vi "recursively populate tree ctl.vi"(8 "error in (no error)":errorcluster, 10 "tree ctl ref":refnum<vi>, 11 "Object path":string="IndivITX/Test1/SA03008N.20190801.000000.itx") -> (0 "error out":errorcluster, 2 "reference out":refnum<vi>)   [LabVIEW 2020, in "Data.S3.lvclass"]
uses:
  Data.S3.lvclass
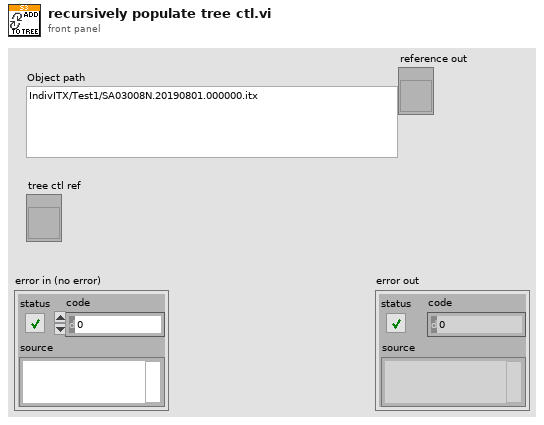
[diagram p1: front panel]
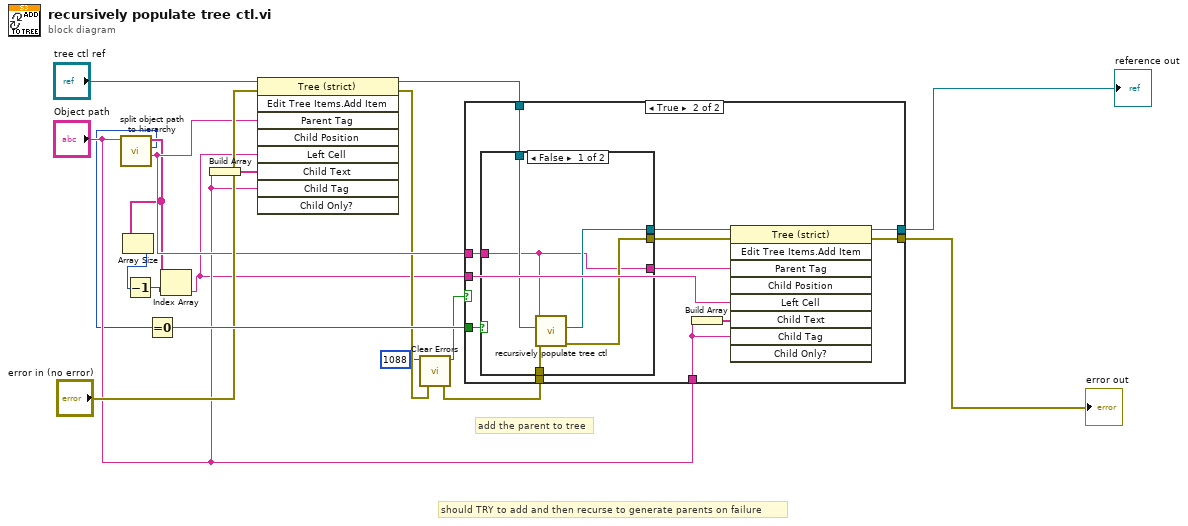
[diagram p0: block diagram]
diagram:
  # "should TRY to add and then recurse to generate parents on failure"
  # "add the parent to tree"
  n1 = call "split object path to hierarchy.vi"("Object path"="Object path") -> ("parent path"=w15:string, "layers"=w2:i32, "hierarchy"=w5:string[])  [unwired: 8 in]
  n2 = Array Size(array=w5) -> (size(s)=w3:i32)
  n3 = Decrement(x=w3) -> (x-1=w4:i32)
  n4 = Equal To 0?(x=w2) -> (x = 0?=w18:bool)
  n5 = Index Array(array=w5, index=w4) -> (element=w1:string)
  n6 = Build Array("Object path") -> (w14:string[])
  n7 = invoke on="Invoke Node" class="Tree (strict)" method="Edit Tree Items.Add Item"(reference="tree ctl ref", error in="error in (no error)", "Parent Tag"=w15, "Left Cell"=w1, "Child Text"=w14, "Child Tag"="Object path") -> (reference out=w12:refnum<vi>, error out=w10:errorcluster)  [unwired: 3 in, 7 out]
  n8 = call <vilib>:"Clear Errors.vi"("error in (no error)"=w10, "specific error code to clear (0: all)"=1088) -> ("error out"=w16:errorcluster, "specific error cleared?"=w9:bool)  [unwired: 4 in]
  n9 = case shown="True" w9 {
    tunnel: [w19 w25] -> w7
    tunnel: w18 -> [_ w32]
    tunnel: [w20 w26] -> w6
    tunnel: w16 -> [w19 w31]
    tunnel: w15 -> [_ w30]
    tunnel: w12 -> [w20 w29]
    tunnel: "Object path" -> [_ w22]
    tunnel: w1 -> [_ w21]
    frame False {
    }
    frame True {
      n10 = case shown="False" w32 {
        tunnel: w31 -> [w37 w40]
        tunnel: w30 -> [w33 w38]
        tunnel: [w34 w40] -> w28
        tunnel: w29 -> [w36 w39]
        tunnel: [w35 w39] -> w27
        tunnel: [w33 w38] -> w24
        frame False {
          n11 = call "recursively populate tree ctl.vi"("error in (no error)"=w37, "tree ctl ref"=w36, "Object path"=w33) -> ("error out"=w34:errorcluster, "reference out"=w35:refnum<vi>)  [unwired: 7 in]
        }
        frame True {
        }
      }
      n12 = Build Array(w22) -> (w23:string[])
      n13 = invoke on="Invoke Node" class="Tree (strict)" method="Edit Tree Items.Add Item"(reference=w27, error in=w28, "Parent Tag"=w24, "Left Cell"=w21, "Child Text"=w23, "Child Tag"=w22) -> (reference out=w26:refnum<vi>, error out=w25:errorcluster)  [unwired: 3 in, 7 out]
    }
  }
  "error out" <- w7
  "reference out" <- w6
